vi "Set Device Property.vi"(0 "Session Handle in":T1, 5 "property":refnum<k21>, 9 "property value":bool, 11 "error in (no error)":errorcluster) -> (4 "Session Handle out":T1, 15 "error out":errorcluster)   [LabVIEW 2015, in "SLSC Switch.lvlib" / "SLSC Session.lvclass"]
uses:
  SLSC Session.lvclass
  Typedefs/Session Handle.ctl
  SLSC Session.lvclass/SLSC Session.ctl
  <vilib>/SLSC/Set Device Property (Bool).vi
  <vilib>/SLSC/SLSC.lvlib
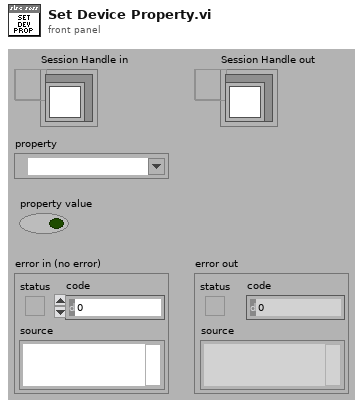
[diagram p1: front panel]
types:
  T1 = typedef "SLSC Switch.lvlib/SLSC Session.lvclass/Session Handle.ctl" = refnum<data-value>
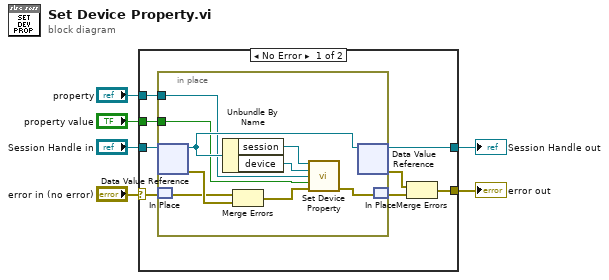
[diagram p0: block diagram]
diagram:
  n1 = case shown="No Error" "error in (no error)" {
    selector: "error in (no error)" -> [w9 w24]
    tunnel: "Session Handle in" -> [w14 w25]
    tunnel: [w13 w25] -> w5
    tunnel: [w10 w24] -> w4
    tunnel: "property" -> [w8 _]
    tunnel: "property value" -> [w7 _]
    frame No Error {
      n2 = in-place {
        in-place-border: w8 -> [w18]
        in-place-border: w7 -> [w17]
        n3 = in-place-dvr #1(w14) -> (w21:refnum<class "SLSC Session.lvclass">, w23:errorcluster)
        n4 = in-place-match #2(w9) -> (w22:errorcluster)
        n5 = Unbundle By Name(w21) -> ("session"=w20:refnum<k21>, "device"=w19:refnum<k21>)
        n6 = Merge Errors(w22, w23) -> (w16:errorcluster)
        n7 = call-poly <vilib>:"Set Device Property.vi"("session in"=w20, "devices"=w19, "property"=w18, "property value"=w17, "error in (no error)"=w16) -> ("error out"=w15:errorcluster)  [unwired: 9 in, 1 out]
        n8 = in-place-dvr #1(w21) -> (w13:T1, w11:errorcluster)
        n9 = in-place-match #2(w15) -> (w12:errorcluster)
      }
      n10 = Merge Errors(w11, w12) -> (w10:errorcluster)
    }
    frame Error {
    }
  }
  "Session Handle out" <- w5
  "error out" <- w4
